vi "Drivetrain Loop.vi"() -> ()   [LabVIEW 2015]
uses:
  Drivetrain Modes.ctl
  Common Code/Change Detect Int.vi
  Robot Global Data.vi
panel:
  out "Mode":T1=enum."Turn to Angle"
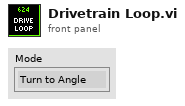
[diagram p1: front panel]
types:
  T1 = typedef "Drivetrain Modes.ctl" = enum16{"Normal", "Cubic Profile", "Trapezoidal Profile", "Turn to Angle", "Distance Drive", "Data Acquisition"}
  T2 = typedef "Drivetrain Commands.ctl" = cluster{"Mode":T1, "Y Power":dbl, "Turn Power":dbl, "Distance":sgl}
  T3 = typedef "WPI_MotorControlDeviceRef.ctl" = cluster{"DeviceStatus":errorcluster, "Type":T4, "PWM":cluster{"PWM Channel":T5, "DeadBand":T6}, "CAN":cluster{"Device Number":u8, "Control Mode":T7, "Semaphore":T8, "Max Vout":dbl, "TalonSRX Control Mode":T9}, "Invert":bool}
  T4 = typedef "WPI_MotorControlType.ctl" = enum16{"PWM", "CAN", "CANTalonSRX"}
  T5 = typedef "FPGA_DIOPWMChannel.ctl" = enum8{"PWM 0", "PWM 1", "PWM 2", "PWM 3", "PWM 4", "PWM 5", "PWM 6", "PWM 7", "PWM 8", "PWM 9", "PWM MXP 0", "PWM MXP 1", "PWM MXP 2", "PWM MXP 3", "PWM MXP 4", "PWM MXP 5", "PWM MXP 6", "PWM MXP 7", "PWM MXP 8", "PWM MXP 9", "Invalid"}
  T6 = typedef "WPI_PWMDeadband.ctl" = cluster{"Name":string, "maxPositivePwm":i32, "minPositivePwm":i32, "centerPwm":i32, "maxNegativePwm":i32, "minNegativePwm":i32, "angularRange":u16}
  T7 = typedef "WPI_CANJaguar_ControlMode.ctl" = enum8{"Percent VBus", "Current", "Speed", "Position", "Voltage"}
  T8 = typedef "Semaphore RefNum" = refnum<k1>
  T9 = typedef "WPI_CANTalonSRX_APIControlMode.ctl" = enum8{"Percent VBus", "Speed", "Position", "Slave", "Unchanged / Invalid"}
  T10 = typedef "Drivetrain Status.ctl" = cluster{"Mode":T1, "Y (Throttle)":dbl, "X (Steer)":dbl, "Trapezoidal Motion Finished?":bool}
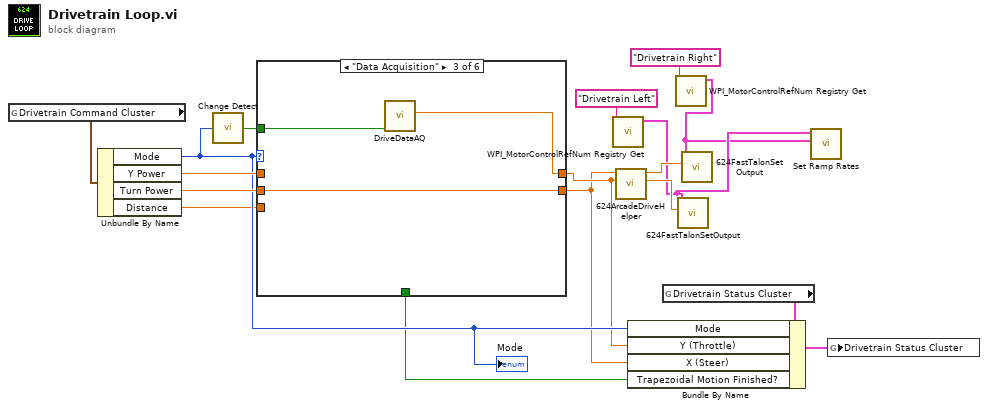
[diagram p0: block diagram]
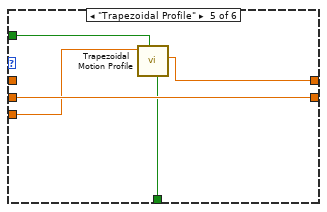
[diagram p5: hidden frame]
diagram:
  n1 = global read "Robot Global Data.vi" "Drivetrain Command Cluster"() -> (w17:T2)
  n2 = Unbundle By Name(w17) -> ("Mode"=w8:T1, "Y Power"=w16:dbl, "Turn Power"=w15:dbl, "Distance"=w3:sgl)
  "Mode" <- w8
  n3 = call-poly "Change Detect.vi"("In"=w8) -> ("Changed?"=w14:bool)
  n4 = case shown="\"Data Acquisition\"" w8 {
    tunnel: w16 -> [_ _ _ w22 _ _]
    tunnel: w15 -> [_ _ w19 w21 w27 _]
    tunnel: w14 -> [_ _ w20 _ w24 _]
    tunnel: [_ _ w18 w22 w26 _] -> w7
    tunnel: [_ _ w19 w21 w27 _] -> w6
    tunnel: [_ _ _ _ w25 _] -> w4
    tunnel: w3 -> [_ _ _ _ w23 _]
    frame "Turn to Angle" {
    }
    frame "Distance Drive" {
    }
    frame "Data Acquisition" {
      n5 = call "DriveDataAQ.vi"("Reset?"=w20) -> ("Throttle Out"=w18:dbl)  [unwired: 10 in]
    }
    frame "Normal", Default {
    }
    frame "Trapezoidal Profile" {
      n6 = call "Trapezoidal Motion Profile.vi"("Reset?"=w24, "Distance"=w23) -> ("Throttle Out"=w26:sgl, "Finished?"=w25:bool)  [unwired: 8 in]
    }
    frame "Cubic Profile" {
    }
  }
  n7 = call <vilib>:"WPI_MotorControlRefNum Registry Get.vi"("refnum name"="Drivetrain Left") -> ("MotorControlDevRef"=w2:T3)  [unwired: 9 in, 1 out]
  n8 = call "624ArcadeDriveHelper.vi"("Y Power"=w7, "Turn Power"=w6) -> ("Left"=w11:dbl, "Right"=w12:dbl)  [unwired: 8 in]
  n9 = global read "Robot Global Data.vi" "Drivetrain Status Cluster"() -> (w9:T10)
  n10 = Bundle By Name(cluster=w9, "Mode"=w8, "Y (Throttle)"=w7, "X (Steer)"=w6, "Trapezoidal Motion Finished?"=w4) -> (w5:T10)
  n11 = call <vilib>:"WPI_MotorControlRefNum Registry Get.vi"("refnum name"="Drivetrain Right") -> ("MotorControlDevRef"=w1:T3)  [unwired: 9 in, 1 out]
  n12 = call "624FastTalonSetOutput.vi"("Output"=w11, "MotorControlDevRef"=w2) -> ()  [unwired: 8 in, 2 out]
  n13 = call "624FastTalonSetOutput.vi"("Output"=w12, "MotorControlDevRef"=w1) -> ()  [unwired: 8 in, 2 out]
  n14 = call "Set Ramp Rates.vi"("DT Right"=w1, "DT Left"=w2) -> ()  [unwired: 10 in]
  n15 = global write "Robot Global Data.vi" "Drivetrain Status Cluster"(w5) -> ()
